vi "3Dto2D.vi"() -> ()   [LabVIEW 2019]
panel:
  in  "Scale":i32=50
  in  "file (use dialog)":path
  out "new picture":picture
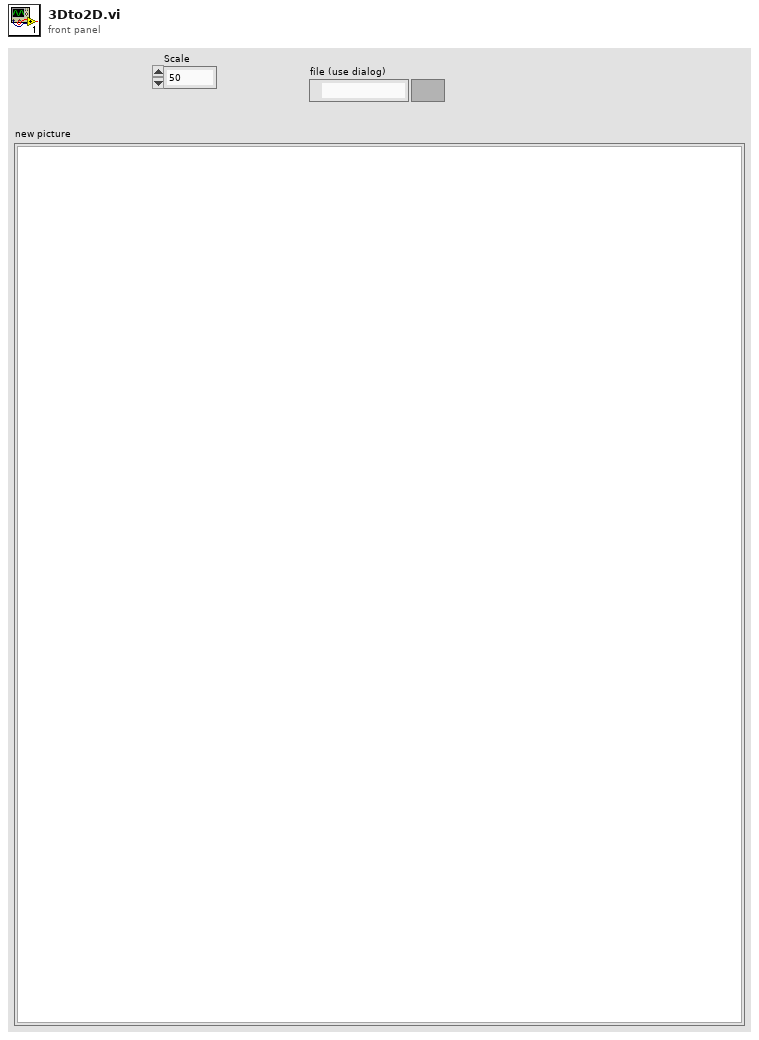
[diagram p1: front panel]
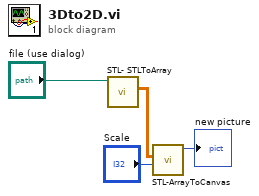
[diagram p0: block diagram]
diagram:
  n1 = call "STL- STLToArray.vi"("file (use dialog)"="file (use dialog)") -> ("Array 3"=w1:dbl[][])  [unwired: 10 in]
  n2 = call "STL-ArrayToCanvas.vi"("Scale"="Scale", "Array 3"=w1) -> ("new picture 3"=→"new picture":picture)  [unwired: 9 in]
